vi "Graph Map.vi"() -> ()   [LabVIEW 2018]
panel:
  in  "Filename":path=path "polarimeter map.lvm"
  out "XY Graph 2":cluster{"Y":dbl[], "Y":dbl[]}[](graph)
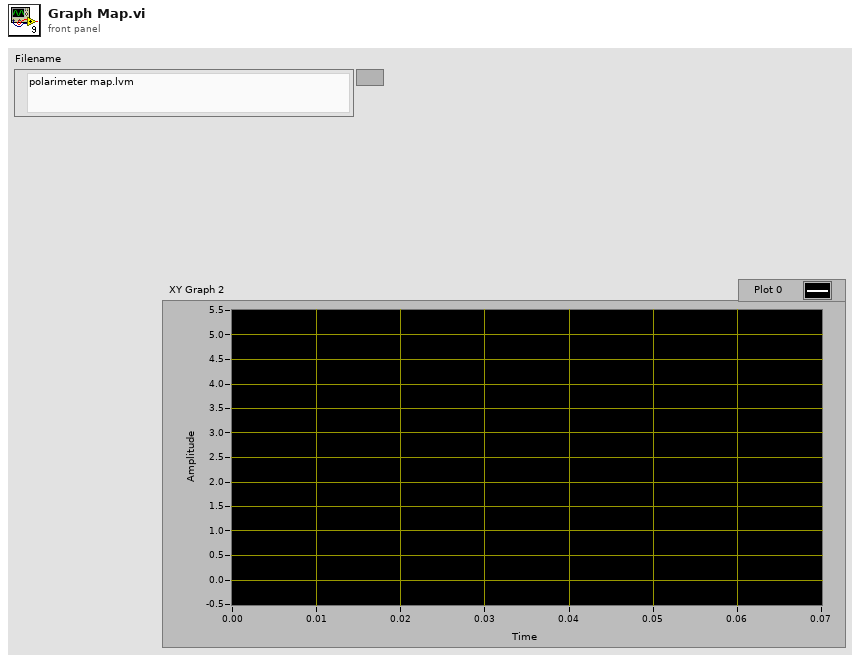
[diagram p1: front panel]
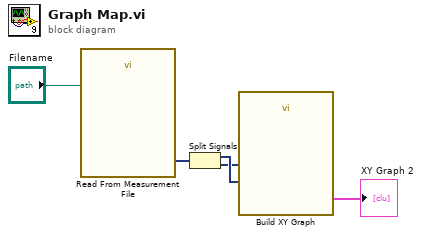
[diagram p0: block diagram]
diagram:
  n1 = call "Read From Measurement File"("Filename"="Filename") -> ("Signals"=w2:dynamicdata)  [unwired: 5 in, 5 out]
  n2 = Split Signals(w2) -> (w4:dynamicdata, w3:dynamicdata)  [unwired: 2 in]
  n3 = call "Build XY Graph"("Y Input"=w4, "X Input"=w3) -> ("XY Graph"=→"XY Graph 2":cluster{"X":dbl[], "Y":dbl[]}[])  [unwired: 8 in, 1 out]
